vi "Run.vi"(7 "Stop Demo":refnum<user-event>, 8 "error in":errorcluster, 9 "Try It Button":refnum<vi>, 10 "Main Subpanel":refnum<vi>, 11 "Interactive in":refnum<class "Interactive.lvclass">) -> (0 "error out":errorcluster, 3 "Interactive out":refnum<class "Interactive.lvclass">)   [LabVIEW 2020, in "Interactive.lvclass"]
uses:
  Interactive.lvclass
  Demo_class/Demo.lvclass
  Interactive.lvclass/Interactive.ctl
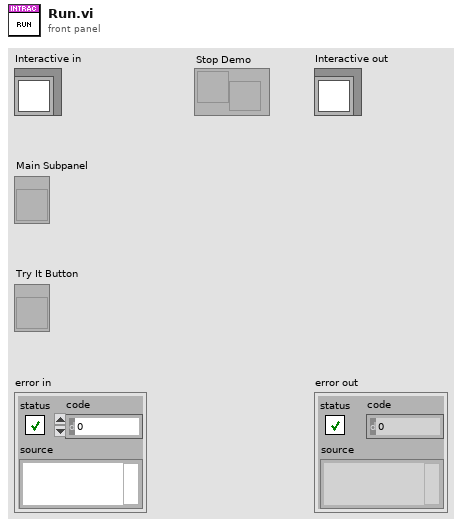
[diagram p1: front panel]
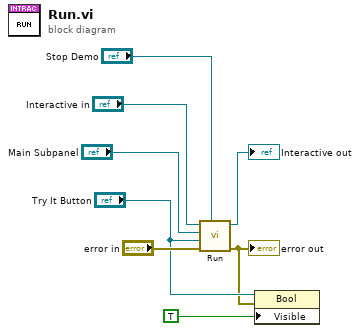
[diagram p0: block diagram]
diagram:
  n1 = call-parent "Run.vi"("Stop Demo"="Stop Demo", "error in"="error in", "Try It Button"="Try It Button", "Main Subpanel"="Main Subpanel", "Demo in"="Interactive in") -> ("error out"=w1:errorcluster, "Demo out"=→"Interactive out":refnum<class "Interactive.lvclass">)  [unwired: 5 in]
  "error out" <- w1
  n2 = property class="Bool"(reference="Try It Button", error in=w1, "Visible"=TRUE) -> ()  [unwired: 2 out]
